vi "Ball_Test.vi"(0 "Left_Joystick_Y":dbl, 1 "X_Button":bool) -> ()   [LabVIEW 2018]
uses:
  Subsytems/Intake_Ball/Intake_Ball_Notifier.ctl
  Subsytems/Intake_Ball/Intake_Ball_Control_Type.ctl
  <vilib>/Rock Robotics/WPI/ThirdParty/Phoenix-LabVIEW/Motor Controller/Controls/CTRE_Phoenix_MotorControl_ControlMode.ctl
  Global_Variables/Intake_Ball_Globals.vi
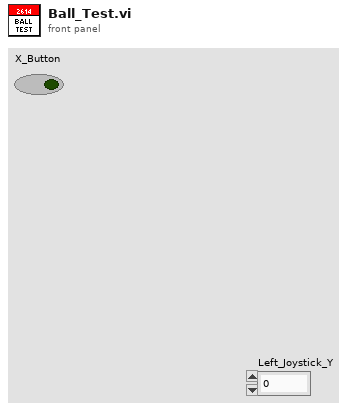
[diagram p1: front panel]
types:
  T1 = typedef "Intake_Ball_Notifier.ctl" = cluster{"Intake_Ball_Control_Type":T2, "Manual_In":bool, "Manual_Out":bool, "Ball_In":bool, "Ball_Out":bool, "Parameter_One":dbl, "Parameter_Two":dbl, "Parameter_Three":dbl, "Step":i32, "Ball_Notifier":refnum<notifier>}
  T2 = typedef "Intake_Ball_Control_Type.ctl" = enum16{"No_Op", "Manual_In", "Manual_Out", "In_Sensor_Stop", "Out_Teleop", "Out", "Stall"}
  T3 = typedef "CTRE_Phoenix_MotorControl_ControlMode.ctl" = u16
  T4 = typedef "WPI_MotorControlDeviceRef.ctl" = cluster{"DeviceStatus":errorcluster, "Type":T5, "PWM":cluster{"PWM Channel":T6, "DeadBand":T7}, "CAN":cluster{"Device Number":u8, "SetOutput VI Ref":variant, "GetOutput VI Ref":variant, "Enable VI Ref":variant, "Disable VI Ref":variant, "Data":variant}, "Invert":bool, "DIO PWM":cluster{"PWM \"Enable\" Channel":T6, "DIOChannel":T8, "PWM Rate":dbl}}
  T5 = typedef "WPI_MotorControlType.ctl" = enum16{"PWM", "CAN", "DIO PWM"}
  T6 = typedef "FPGA_DIOPWMChannel.ctl" = enum8{"PWM 0", "PWM 1", "PWM 2", "PWM 3", "PWM 4", "PWM 5", "PWM 6", "PWM 7", "PWM 8", "PWM 9", "PWM MXP 0", "PWM MXP 1", "PWM MXP 2", "PWM MXP 3", "PWM MXP 4", "PWM MXP 5", "PWM MXP 6", "PWM MXP 7", "PWM MXP 8", "PWM MXP 9", "Invalid"}
  T7 = typedef "WPI_PWMDeadband.ctl" = cluster{"Name":string, "maxPositivePwm":i32, "minPositivePwm":i32, "centerPwm":i32, "maxNegativePwm":i32, "minNegativePwm":i32, "angularRange":u16}
  T8 = typedef "FPGA_DIOChannel.ctl" = enum8{"DIO 0", "DIO 1", "DIO 2", "DIO 3", "DIO 4", "DIO 5", "DIO 6", "DIO 7", "DIO 8", "DIO 9", "DIO MXP 0", "DIO MXP 1", "DIO MXP 2", "DIO MXP 3", "DIO MXP 4", "DIO MXP 5", "DIO MXP 6", "DIO MXP 7", "DIO MXP 8", "DIO MXP 9", "DIO MXP 10", "DIO MXP 11", "DIO MXP 12", "DIO MXP 13", "DIO MXP 14", "DIO MXP 15", "SPI Port CS1", "SPI Port CS2", "SPI Port CS3", "SPI Port MISO", "SPI Port MOSI", "Invalid"}
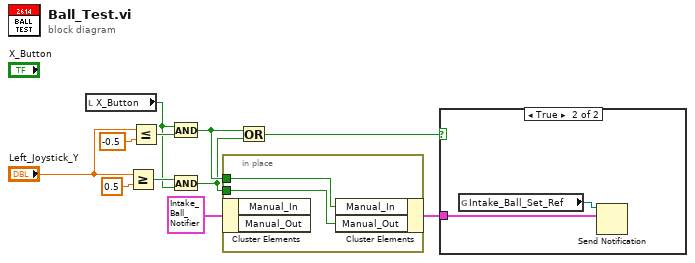
[diagram p0: block diagram]
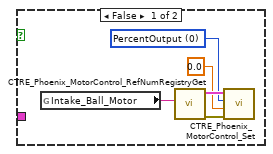
[diagram p2: hidden frame]
diagram:
  n1 = local read "X_Button"() -> (w4:bool)
  n2 = Greater Or Equal?(x="Left_Joystick_Y", y=0.5) -> (x >= y?=w6:bool)
  n3 = Less Or Equal?(x="Left_Joystick_Y", y=-0.5) -> (x <= y?=w5:bool)
  n4 = And(x=w4, y=w5) -> (x .and. y?=w3:bool)
  n5 = And(x=w6, y=w4) -> (x .and. y?=w2:bool)
  n6 = in-place {
    in-place-border: w2 -> [w12]
    in-place-border: w3 -> [w13]
    n7 = in-place-cluster #1(T1 {"Intake_Ball_Control_Type"=enum."No_Op", "Manual_In"=FALSE, "Manual_Out"=FALSE, "Ball_In"=FALSE, "Ball_Out"=FALSE, "Parameter_One"=0.0, "Parameter_Two"=0.0, "Parameter_Three"=0.0, "Step"=0, "Ball_Notifier"=refnum} ("Intake_Ball_Notifier")) -> ()  [unwired: 2 out]
    n8 = in-place-cluster #1("Manual_In"=w13, "Manual_Out"=w12) -> (w11:T1)
  }
  n9 = Or(x=w3, y=w2) -> (x .or. y?=w1:bool)
  n10 = case shown="True" w1 {
    tunnel: w11 -> [_ w20]
    frame False {
      w14 = T3 0 items=["PercentOutput"=0, "Position"=1, "Velocity"=2, "Current"=3, "Follower"=5, "MotionProfile"=6, "MotionMagic"=7, "MotionProfileArc"=10, "Disabled"=15] ("Control Mode")
      n11 = global read "Intake_Ball_Globals.vi" "Intake_Ball_Motor"() -> (w18:string)
      n12 = call <vilib>:"CTRE_Phoenix_MotorControl_RefNumRegistryGet.vi"("refnum name"=w18) -> ("error out"=w16:errorcluster, "PhoenixMotorControlDevRef"=w17:T4)  [unwired: 9 in]
      n13 = call <vilib>:"CTRE_Phoenix_MotorControl_Set.vi"("error in (no error)"=w16, "Output"=0.0, "Control Mode"=w14, "PhoenixMotorControlDevRef"=w17) -> ()  [unwired: 6 in, 2 out]
    }
    frame True {
      n14 = global read "Intake_Ball_Globals.vi" "Intake_Ball_Set_Ref"() -> (w19:refnum<notifier>)
      n15 = Send Notification(notification=w20, notifier=w19) -> ()  [unwired: 1 in, 2 out]
    }
  }
